vi "1Gear.vi"(8 "2 Gear Side":enum16{"Left", "Right"}(ring), 9 "2 Gear":bool, 10 "Gear Side":enum16{"Center", "Left", "Right"}(ring), 11 "RobotDriveDevRef":T1={"DevStatus"={"status"=FALSE, "code"=0, "source"=""}, "Motors[]"=[], "Square Inputs"=FALSE, "Max Output"=1.0}) -> (3 "RobotDriveDevRef":T1={"DevStatus"={"status"=FALSE, "code"=0, "source"=""}, "Motors[]"=[], "Square Inputs"=FALSE, "Max Output"=1.0})   [LabVIEW 2016]
uses:
  <vilib>/Rock Robotics/WPI/RobotDrive/WPI_RobotDriveDevRef.ctl
  <vilib>/Rock Robotics/WPI/MotorControl/WPI_MotorControlDeviceRef.ctl
  <vilib>/Rock Robotics/WPI/MotorControl/WPI_MotorControlType.ctl
  <vilib>/Rock Robotics/SystemInterfaces/DIO/FPGA_DIOPWMChannel.ctl
  <vilib>/Rock Robotics/WPI/PWM/WPI_PWMDeadband.ctl
  <vilib>/Rock Robotics/WPI/RobotDrive/WPI_RobotDriveArcadeDrive_Standard(NoSaturation).vi
  Robot Global Data.vi
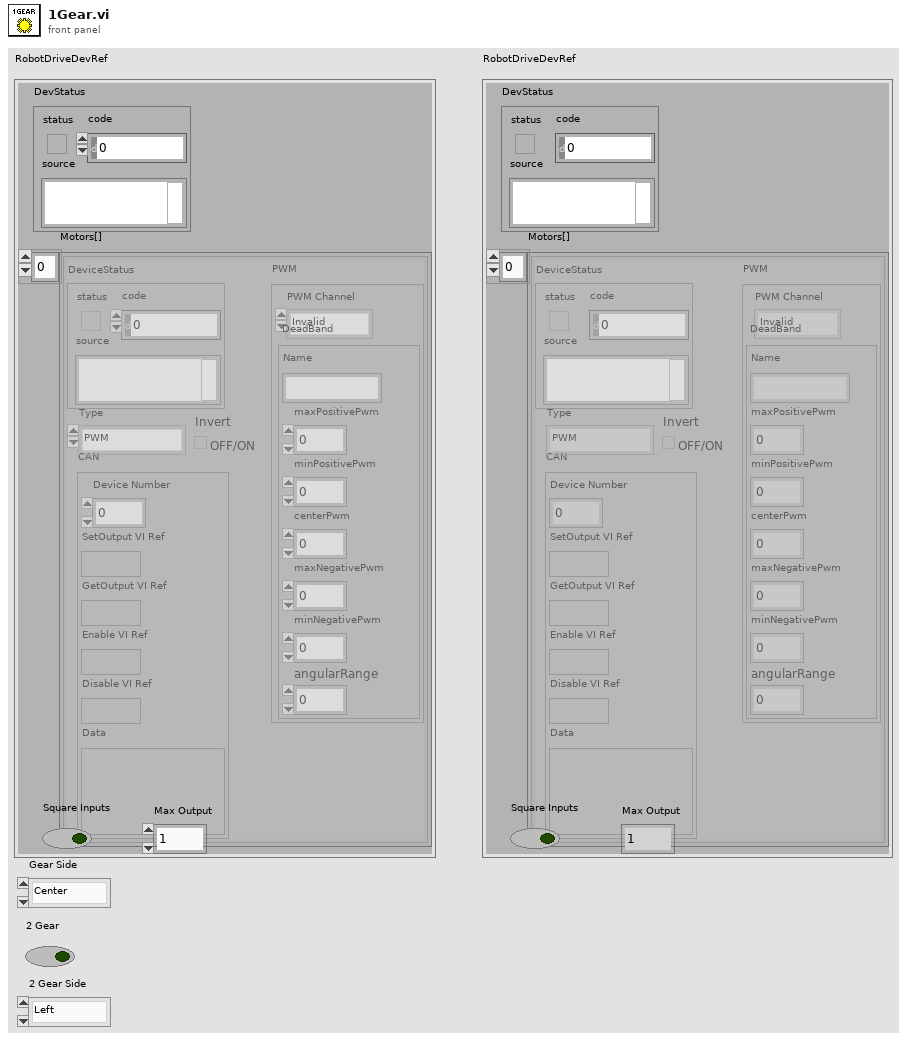
[diagram p1: front panel]
types:
  T1 = typedef "WPI_RobotDriveDevRef.ctl" = cluster{"DevStatus":errorcluster, "Motors[]":T2[], "Square Inputs":bool, "Max Output":dbl}
  T2 = typedef "WPI_MotorControlDeviceRef.ctl" = cluster{"DeviceStatus":errorcluster, "Type":T3, "PWM":cluster{"PWM Channel":T4, "DeadBand":T5}, "CAN":cluster{"Device Number":u8, "SetOutput VI Ref":variant, "GetOutput VI Ref":variant, "Enable VI Ref":variant, "Disable VI Ref":variant, "Data":variant}, "Invert":bool}
  T3 = typedef "WPI_MotorControlType.ctl" = enum16{"PWM", "CAN"}
  T4 = typedef "FPGA_DIOPWMChannel.ctl" = enum8{"PWM 0", "PWM 1", "PWM 2", "PWM 3", "PWM 4", "PWM 5", "PWM 6", "PWM 7", "PWM 8", "PWM 9", "PWM MXP 0", "PWM MXP 1", "PWM MXP 2", "PWM MXP 3", "PWM MXP 4", "PWM MXP 5", "PWM MXP 6", "PWM MXP 7", "PWM MXP 8", "PWM MXP 9", "Invalid"}
  T5 = typedef "WPI_PWMDeadband.ctl" = cluster{"Name":string, "maxPositivePwm":i32, "minPositivePwm":i32, "centerPwm":i32, "maxNegativePwm":i32, "minNegativePwm":i32, "angularRange":u16}
  T6 = cluster{"Lower X":dbl, "Lower Y":dbl, "Upper X":dbl, "Upper Y":dbl, "Lower Limit":dbl, "Upper Limit":dbl}
  T7 = cluster{"Target?":bool, "PegAngle":dbl, "Distance":dbl}
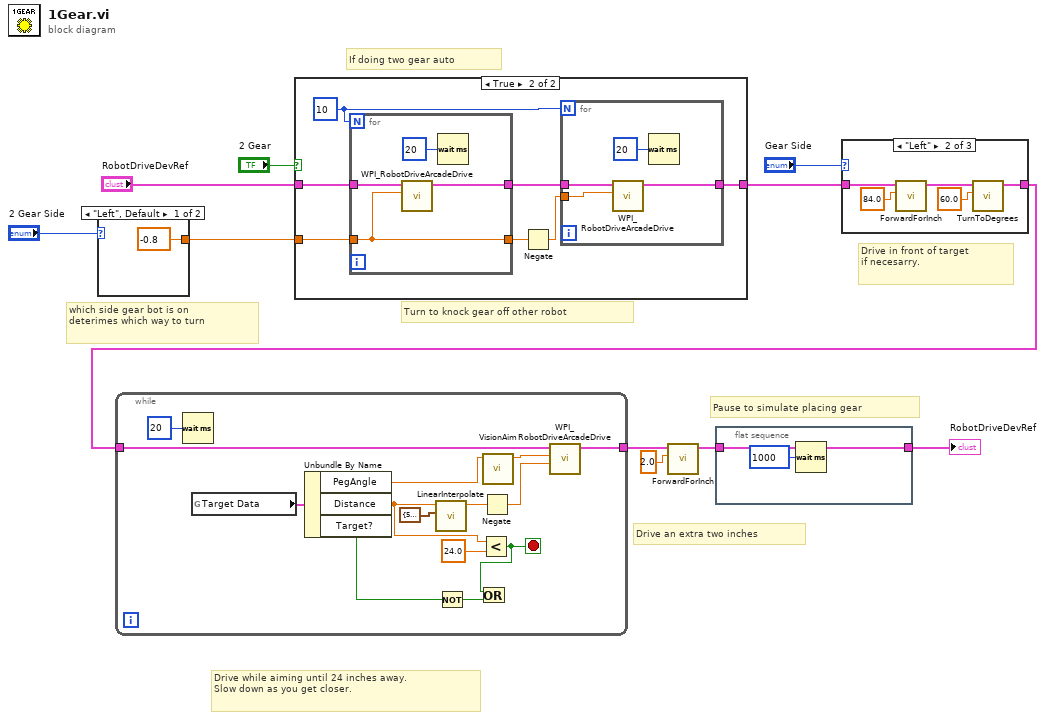
[diagram p0: block diagram]
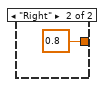
[diagram p2: hidden frame]
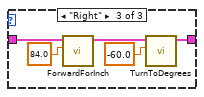
[diagram p5: hidden frame]
diagram:
  # "If doing two gear auto"
  # "Pause to simulate placing gear"
  # "Drive an extra two inches"
  # "Drive while aiming until 24 inches away.\nSlow down as you get closer."
  # "Drive in front of target\nif necesarry."
  # "which side gear bot is on\ndeterimes which way to turn"
  # "Turn to knock gear off other robot"
  n1 = case shown="\"Left\", Default" "2 Gear Side" {
    tunnel: [-0.8 ("X axis value") 0.8 ("X axis value")] -> w5
    frame "Left", Default {
    }
    frame "Right" {
    }
  }
  n2 = case shown="True" "2 Gear" {
    tunnel: "RobotDriveDevRef" -> [w14 w21]
    tunnel: [w14 w18] -> w7
    tunnel: w5 -> [_ w15]
    frame False {
    }
    frame True {
      w20 = 10
      n3 = for {
        N: w20 -> [_]
        tunnel: w21 -> [w29]
        tunnel: [w27] -> w19
        tunnel: [w26] -> w17
        tunnel: w15 -> [w26]
        n4 = call-poly <vilib>:"WPI_RobotDriveArcadeDrive.vi"("X axis value"=w26, "RobotDriveDevRef"=w29) -> ("RobotDriveDevRef"=w27:T1)  [unwired: 7 in, 2 out]
        n5 = Wait (ms)(milliseconds to wait=u32 20) -> ()  [unwired: 1 out]
      }
      n6 = Negate(x=w17) -> (-x=w16:dbl)
      n7 = for {
        N: w20 -> [_]
        tunnel: w19 -> [w25]
        tunnel: [w23] -> w18
        tunnel: w16 -> [w22]
        n8 = call-poly <vilib>:"WPI_RobotDriveArcadeDrive.vi"("X axis value"=w22, "RobotDriveDevRef"=w25) -> ("RobotDriveDevRef"=w23:T1)  [unwired: 7 in, 2 out]
        n9 = Wait (ms)(milliseconds to wait=u32 20) -> ()  [unwired: 1 out]
      }
    }
  }
  n10 = flat-sequence {
    tunnel: w2 -> [w31]
    tunnel: [w31] -> w1
    frame #0 {
      n11 = Wait (ms)(milliseconds to wait=u32 1000) -> ()  [unwired: 1 out]
    }
  }
  n12 = case shown="\"Left\"" "Gear Side" {
    tunnel: [w32 w36 w41] -> w3
    tunnel: w7 -> [w32 w35 w40]
    frame "Center", Default {
    }
    frame "Left" {
      n13 = call "ForwardForInch.vi"("Distance"=84.0, "RobotDriveDevRef"=w35) -> ("RobotDriveDevRef 2"=w37:T1)  [unwired: 9 in]
      n14 = call "TurnToDegrees.vi"("Angle"=60.0, "RobotDriveDevRef"=w37) -> ("RobotDriveDevRef 2"=w36:T1)  [unwired: 9 in]
    }
    frame "Right" {
      n15 = call "ForwardForInch.vi"("Distance"=84.0, "RobotDriveDevRef"=w40) -> ("RobotDriveDevRef 2"=w42:T1)  [unwired: 9 in]
      n16 = call "TurnToDegrees.vi"("Angle"=-60.0, "RobotDriveDevRef"=w42) -> ("RobotDriveDevRef 2"=w41:T1)  [unwired: 9 in]
    }
  }
  n17 = while {
    tunnel: [w56] -> w11
    tunnel: w3 -> [w46]
    stop <- w43 stop-if-true
    n18 = Wait (ms)(milliseconds to wait=u32 20) -> ()  [unwired: 1 out]
    n19 = global read "Robot Global Data.vi" "Target Data"() -> (w52:T7)
    n20 = Unbundle By Name(w52) -> ("PegAngle"=w51:dbl, "Distance"=w47:dbl, "Target?"=w44:bool)
    n21 = call "LinearInterpolate.vi"("Config"=T6 {"Lower X"=55.0, "Lower Y"=0.48, "Upper X"=65.0, "Upper Y"=0.8, "Lower Limit"=0.45, "Upper Limit"=0.75}, "Value"=w47) -> ("Ouput"=w48:dbl)  [unwired: 9 in]
    n22 = Not(x=w44) -> (.not. x?=w45:bool)
    n23 = Less?(x=w47, y=24.0) -> (x < y?=w43:bool)
    n24 = Or(x=w43, y=w45) -> ()  [unwired: 1 out]
    n25 = Negate(x=w48) -> (-x=w53:dbl)
    n26 = call "VisionAim.vi"("Angle"=w51) -> ("Turn Amount"=w49:dbl)  [unwired: 9 in, 1 out]
    n27 = call-poly <vilib>:"WPI_RobotDriveArcadeDrive.vi"("Y axis value"=w53, "X axis value"=w49, "RobotDriveDevRef"=w46) -> ("RobotDriveDevRef"=w56:T1)  [unwired: 6 in, 2 out]
  }
  n28 = call "ForwardForInch.vi"("Distance"=2.0, "RobotDriveDevRef"=w11) -> ("RobotDriveDevRef 2"=w2:T1)  [unwired: 9 in]
  "RobotDriveDevRef" <- w1
